vi "Serialize.vi"(0 "Input 6":variant, 4 "Input 5":variant, 6 "Input 4":variant, 8 "Input 3":variant, 9 "Input 2":variant, 10 "Input 1":variant, 11 "Actor in":refnum<class "Actor.lvclass">) -> (3 "Actor out":refnum<class "Actor.lvclass">)   [LabVIEW 2021, in "jettl.lvlib" / "Actor.lvlib" / "Actor.lvclass"]
uses:
  Actor.lvclass
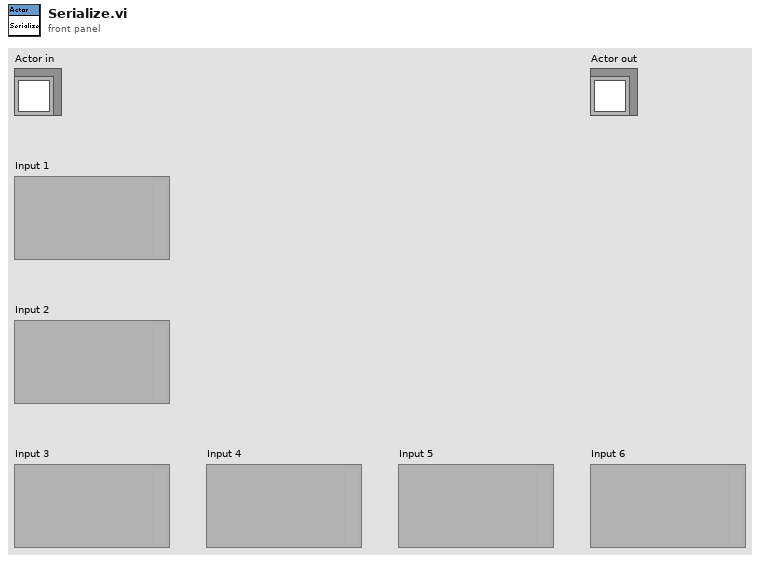
[diagram p1: front panel]
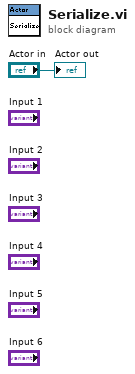
[diagram p0: block diagram]
diagram:
  "Actor out" <- "Actor in"
